vi "n load cor.vi"(8 "error in (no error)":errorcluster, 10 "filename":string, 11 "n":u16) -> (0 "error out":errorcluster, 3 "function return":i16)   [LabVIEW 2015, in "SCANalone4x64.lvlib"]
doc: "__declspec(dllimport) short __stdcall n_load_cor(unsigned short n, const char* filename);"
uses:
  <userlib>/SCANalone4x64/SCANalone4x64.lvlib
  <userlib>/SCANalone4x64/SCANalone4x64.dll
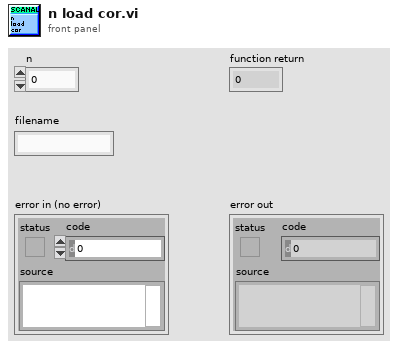
[diagram p1: front panel]
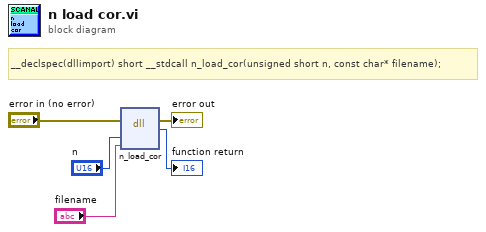
[diagram p0: block diagram]
diagram:
  # "__declspec(dllimport) short __stdcall n_load_cor(unsigned short n, const char* filename);"
  n1 = dll-call lib="C:/Program Files/National Instruments/LabVIEW 2015/user.lib/SCANalone4x64/SCANalone4x64.*" fn="n_load_cor"(error in="error in (no error)", "n"="n", "filename"="filename") -> (error out=→"error out":errorcluster, →"function return":i16)  [unwired: 4 in, 1 out]
